vi "Default Instrument Setup.vi"(8 "error in (no error)":errorcluster, 11 "VISA resource name":refnum<visa-resource-name>) -> (0 "error out":errorcluster, 3 "VISA resource name out":refnum<visa-resource-name>)   [LabVIEW 2021, in "Yokogawa WT1800 Series.lvlib"]
doc: "This Utility VI sends a default command string to the instrument whenever a new VISA session is opened, or the instrument is reset. Use this VI as a subVI for the <B>Initialize</B> and <B>Reset</B> VIs. Altering this VI could cause these two VIs to operate incorrectly."
uses:
  <instrlib>/Yokogawa WT1800 Series/Yokogawa WT1800 Series.lvlib
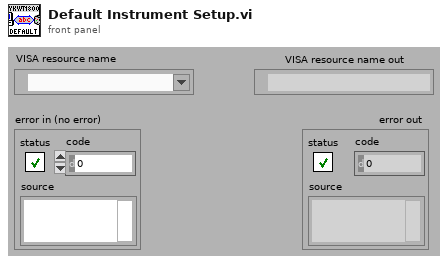
[diagram p1: front panel]
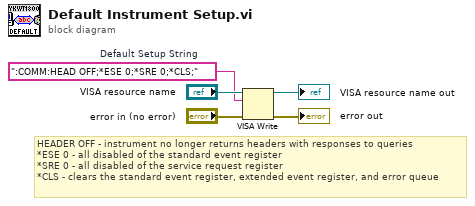
[diagram p0: block diagram]
diagram:
  w1 = ":COMM:HEAD OFF;*ESE 0;*SRE 0;*CLS;"  # Default Setup String
  # "HEADER OFF - instrument no longer returns headers with responses to queries\n*ESE 0 - all disabled of the standard event register\n*SRE 0 - all disabled of the service request register\n*CLS - clears the standard event register, extended event register, and error queue"
  n1 = VISA Write(VISA resource name="VISA resource name", write buffer=w1, error in (no error)="error in (no error)") -> (VISA resource name out=→"VISA resource name out":refnum<visa-resource-name>, error out=→"error out":errorcluster)  [unwired: 1 out]
